vi "Serial Test Bench.vi"() -> ()   [LabVIEW 2017]
uses:
  Controls/Rigid Body Info.ctl
  Controls/Position.ctl
  Controls/Orientation.ctl
  Controls/Tracker Type.ctl
  Controls/COM Port.ctl
  Controls/Tracking Data.ctl
  Controls/Packet Data.ctl
panel:
  in  "Aurora COM Port":T1=enum."COM4"
  in  "Tracker":T2
  out "error out":errorcluster
  in  "error in (no error)":errorcluster
  out "Rigid Body Data":T3
  in  "stop":bool
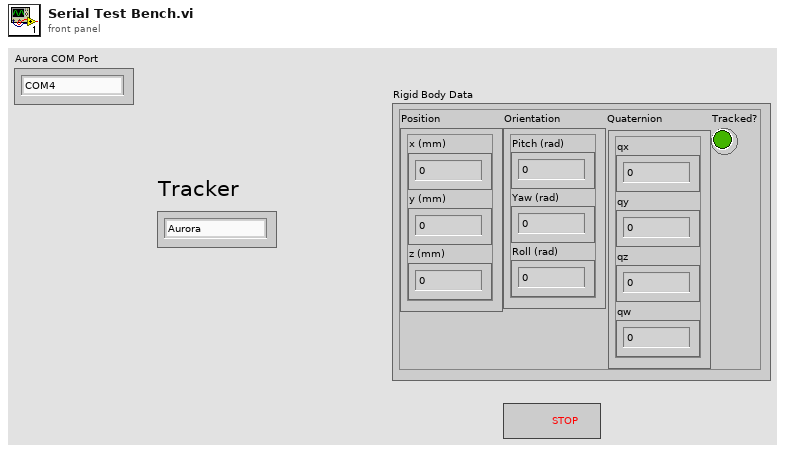
[diagram p1: front panel]
types:
  T1 = typedef "COM Port.ctl" = enum16{"COM1", "COM2", "COM3", "COM4", "COM5", "COM6", "COM7", "COM8", "COM9", "COM10"}
  T2 = typedef "Tracker Type.ctl" = enum16{"Aurora", "OptiTrack"}
  T3 = typedef "Rigid Body Info.ctl" = cluster{"Position":T4, "Orientation":T5, "Quaternion":cluster{"qx":sgl, "qy":sgl, "qz":sgl, "qw":sgl}, "Tracked?":bool}
  T4 = typedef "Position.ctl" = cluster{"x (mm)":sgl, "y (mm)":sgl, "z (mm)":sgl}
  T5 = typedef "Orientation.ctl" = cluster{"Pitch (rad)":sgl, "Yaw (rad)":sgl, "Roll (rad)":sgl}
  T6 = typedef "Tracking Data.ctl" = cluster{"VISA resource name":refnum<visa-resource-name>, "Packet Data":T7, "Rigid Body Data":T3, "Position Array":dbl[][], "Tracker":T2}
  T7 = typedef "Packet Data.ctl" = cluster{"Frame Number (UINT32)":u32, "Number of Rigid Bodies (UINT32)":u32, "Timestamp (double float)":dbl}
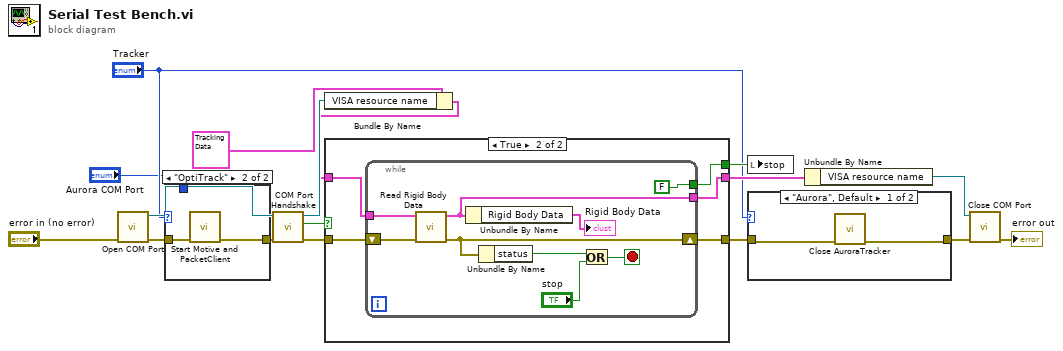
[diagram p0: block diagram]
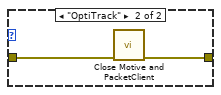
[diagram p2: hidden frame]
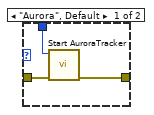
[diagram p3: hidden frame]
diagram:
  n1 = call "Open COM Port.vi"("error in (no error)"="error in (no error)") -> ("error out"=w12:errorcluster, "VISA Refnum out"=w8:refnum<visa-resource-name>)  [unwired: 9 in]
  n2 = case shown="\"OptiTrack\"" "Tracker" {
    tunnel: w12 -> [w19 w22]
    tunnel: [w20 w21] -> w11
    tunnel: "Aurora COM Port" -> [w18 _]
    frame "Aurora", Default {
      n3 = call "Start AuroraTracker.vi"("Error In"=w19, "Aurora COM Port"=w18) -> ("Error Out"=w20:errorcluster)  [unwired: 9 in]
    }
    frame "OptiTrack" {
      n4 = call "Start Motive and PacketClient.vi"("Error In"=w22) -> ("Error Out"=w21:errorcluster)  [unwired: 10 in]
    }
  }
  n5 = call "COM Port Handshake.vi"("error in (no error)"=w11, "VISA Refnum in"=w8) -> ("error out"=w16:errorcluster, "OptiTrack Connected?"=w15:bool, "VISA Refnum out"=w7:refnum<visa-resource-name>)  [unwired: 7 in]
  n6 = Bundle By Name(cluster=T6 {"VISA resource name"="", "Packet Data"={"Frame Number (UINT32)"=0, "Number of Rigid Bodies (UINT32)"=0, "Timestamp (double float)"=0.0}, "Rigid Body Data"={"Position"={"x (mm)"=0.0, "y (mm)"=0.0, "z (mm)"=0.0}, "Orientation"={"Pitch (rad)"=0.0, "Yaw (rad)"=0.0, "Roll (rad)"=0.0}, "Quaternion"={"qx"=0.0, "qy"=0.0, "qz"=0.0, "qw"=0.0}, "Tracked?"=FALSE}, "Position Array"=[], "Tracker"=enum."Aurora"} ("Tracking Data In"), "VISA resource name"=w7) -> (w2:T6)
  n7 = case shown="True" w15 {
    selector: w15 -> [w24 _]
    tunnel: [w24 w30] -> w17
    tunnel: w2 -> [w23 w29]
    tunnel: w16 -> [w25 w28]
    tunnel: [w23 w27] -> w5
    tunnel: [w25 w26] -> w10
    frame False {
    }
    frame True {
      n8 = while {
        shift-right: [w33] -> w26
        shift-left: w28 -> [w39]
        tunnel: [w32] -> w27
        tunnel: w29 -> [w35]
        tunnel: [FALSE] -> w30
        stop <- w36 stop-if-true
        n9 = call "Read Rigid Body Data.vi"("error in (no error)"=w39, "Tracking Data In"=w35) -> ("error out"=w33:errorcluster, "Tracking Data Out"=w32:T6)  [unwired: 8 in]
        n10 = Unbundle By Name(w32) -> ("Rigid Body Data"=→"Rigid Body Data":T3)
        n11 = Unbundle By Name(w33) -> ("status"=w38:bool)
        n12 = Or(x=w38, y="stop") -> (x .or. y?=w36:bool)
      }
    }
  }
  n13 = local write "stop"(w17) -> ()
  n14 = case shown="\"Aurora\", Default" "Tracker" {
    tunnel: w10 -> [w41 w43]
    tunnel: [w40 w42] -> w9
    frame "Aurora", Default {
      n15 = call "Close AuroraTracker.vi"("Error In"=w41) -> ("Error Out"=w40:errorcluster)  [unwired: 10 in]
    }
    frame "OptiTrack" {
      n16 = call "Close Motive and PacketClient.vi"("Error In"=w43) -> ("Error Out"=w42:errorcluster)  [unwired: 10 in]
    }
  }
  n17 = Unbundle By Name(w5) -> ("VISA resource name"=w4:refnum<visa-resource-name>)
  n18 = call "Close COM Port.vi"("error in (no error)"=w9, "VISA Refnum in"=w4) -> ("error out"=→"error out":errorcluster)  [unwired: 9 in]
